vi "Get Inspection Limits.vi"(8 "error in (no error)":errorcluster, 10 "dummy":bool) -> (0 "error out":errorcluster, 1 "timed out?":bool, 2 "Reply Payload":T1={"MaxSamples"=50800, "PosToStartScan"=50800, "PosToEndScan"=0, "ScanLength"=50800})   [LabVIEW 2015, in "Tool Module.lvlib"]
doc: "Get the values for the inspection axial limits plus max samples.\n_____\nCreated using Delacor QMH Event Scripter 2.1.0.3."
uses:
  Tool Module.lvlib
  Get Inspection Limits (Reply Payload)--cluster.ctl
  Get Inspection Limits Argument--cluster.ctl
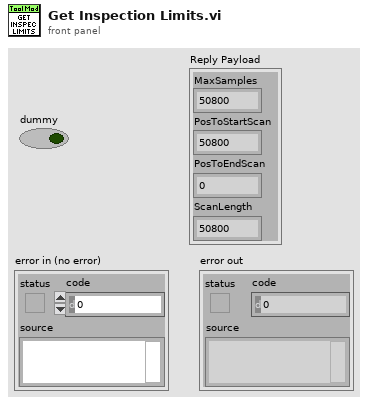
[diagram p1: front panel]
types:
  T1 = typedef "Tool Module.lvlib/Get Inspection Limits (Reply Payload)--cluster.ctl" = cluster{"MaxSamples":i32, "PosToStartScan":i32, "PosToEndScan":i32, "ScanLength":i32}
  T2 = typedef "Tool Module.lvlib/Get Inspection Limits Argument--cluster.ctl" = cluster{"dummy":bool, "Wait Notifier":refnum<notifier>}
  T3 = typedef "Tool Module.lvlib/Request Events--cluster.ctl" = cluster{"Stop Module":refnum<user-event>, "Show Panel":refnum<user-event>, "Hide Panel":refnum<user-event>, "Get Module Execution Status":refnum<user-event>, "Show Diagram":refnum<user-event>, "Test Trig 2":refnum<user-event>, "GOTO":refnum<user-event>, "Start Inspect":refnum<user-event>, "CONNECT":refnum<user-event>, "Get All Inspect Data":refnum<user-event>, "Get Inspection Limits":refnum<user-event>, "Set Inspection Limits":refnum<user-event>, "Update Status":refnum<user-event>, "Get Data Format Params":refnum<user-event>, "Start Data Monitor":refnum<user-event>, "Get FPGA Setup Params":refnum<user-event>, "Set FPGA Setup Params":refnum<user-event>, "Set Tool Config":refnum<user-event>, "Get Tool Config":refnum<user-event>, "Set Integration Count":refnum<user-event>, "Set Laser Params":refnum<user-event>, "Get Mtrl Ctrl Reg":refnum<user-event>, "Commit Ctrl Reg":refnum<user-event>, "Set Event Logger":refnum<user-event>, "Write to File":refnum<user-event>, "Read from File":refnum<user-event>, "Set Device Temp Thresholds":refnum<user-event>}
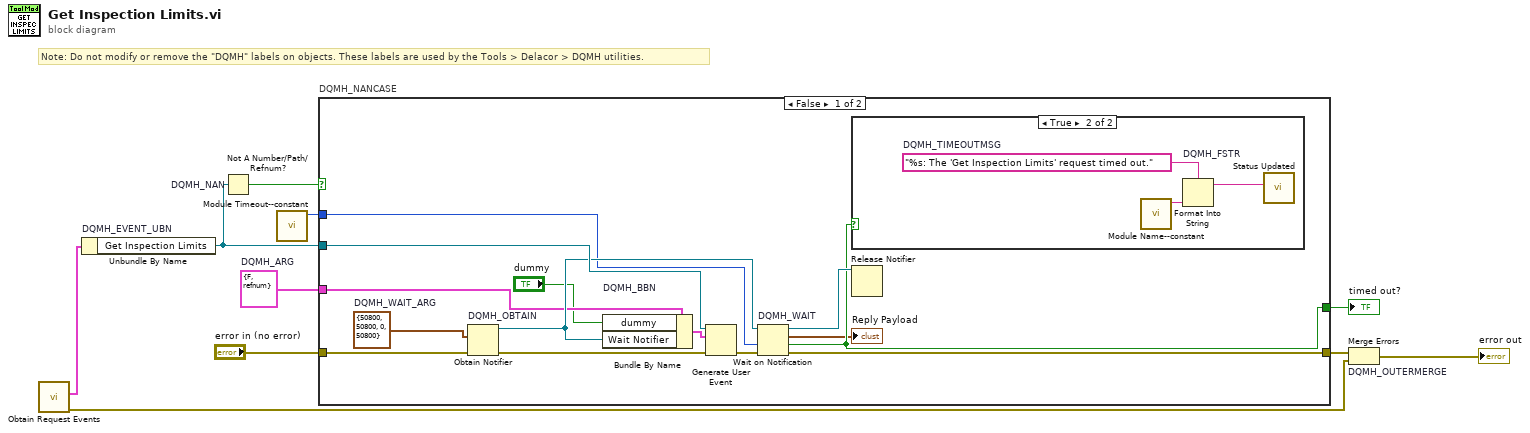
[diagram p0: block diagram]
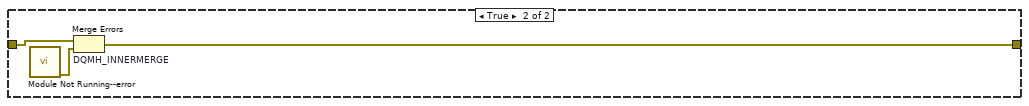
[diagram p3: hidden frame]
diagram:
  w4 = T2 {"dummy"=FALSE, "Wait Notifier"=refnum}  # DQMH_ARG
  # "Note: Do not modify or remove the \"DQMH\" labels on objects. These labels are used by the Tools > Delacor > DQMH utilities."
  n1 = call "Obtain Request Events.vi"() -> ("error out"=w2:errorcluster, "Tool Module Request Events"=w1:T3)  [unwired: 10 in]
  n2 = Unbundle By Name "DQMH_EVENT_UBN"(w1) -> ("Get Inspection Limits"=w8:refnum<user-event>)
  n3 = Not A Number/Path/Refnum? "DQMH_NAN"(number/path/refnum=w8) -> (NaN/Path/Refnum?=w7:bool)
  n4 = call "Module Timeout--constant.vi"() -> ("Module Timeout"=w3:i32)  [unwired: 11 in]
  n5 = case "DQMH_NANCASE" shown="False" w7 {
    tunnel: "error in (no error)" -> [w24 w30]
    tunnel: w8 -> [w22 _]
    tunnel: [w18 w29] -> w5
    tunnel: [w15 _] -> w6
    tunnel: w4 -> [w14 _]
    tunnel: w3 -> [w12 _]
    frame False {
      w19 = T1 {"MaxSamples"=50800, "PosToStartScan"=50800, "PosToEndScan"=0, "ScanLength"=50800}  # DQMH_WAIT_ARG
      n6 = Obtain Notifier "DQMH_OBTAIN"(notification data type=w19, error in (no error)=w24) -> (notifier out=w17:refnum<notifier>, error out=w20:errorcluster)  [unwired: 2 in, 1 out]
      n7 = Bundle By Name "DQMH_BBN"(cluster=w14, "dummy"="dummy", "Wait Notifier"=w17) -> (w21:T2)
      n8 = Generate User Event(user event=w22, event data cluster=w21, error in=w20) -> (error out=w23:errorcluster)  [unwired: 1 in, 1 out]
      n9 = Wait on Notification "DQMH_WAIT"(notifier=w17, timeout in ms (-1)=w12, error in (no error)=w23) -> (notifier out=w16:refnum<notifier>, notification=→"Reply Payload":T1, timed out?=w15:bool, error out=w18:errorcluster)  [unwired: 1 in]
      n10 = case shown="True" w15 {
        frame False {
        }
        frame True {
          w27 = "%s: The 'Get Inspection Limits' request timed out."  # DQMH_TIMEOUTMSG
          n11 = call "Module Name--constant.vi"() -> ("Module Name"=w26:string)  [unwired: 11 in]
          n12 = Format Into String "DQMH_FSTR"(format string=w27, w26) -> (resulting string=w25:string)  [unwired: 2 in, 1 out]
          n13 = call "Status Updated.vi"("Status"=w25) -> ()  [unwired: 10 in, 1 out]
        }
      }
      n14 = Release Notifier(notifier=w16) -> ()  [unwired: 2 in, 3 out]
    }
    frame True {
      n15 = call "Module Not Running--error.vi"() -> ("error out"=w28:errorcluster)  [unwired: 11 in]
      n16 = Merge Errors "DQMH_INNERMERGE"(w30, w28) -> (w29:errorcluster)
    }
  }
  "timed out?" <- w6
  n17 = Merge Errors "DQMH_OUTERMERGE"(w5, w2) -> (→"error out":errorcluster)
